vi "unused_getType.vi"(8 "error in (no error)":errorcluster, 11 "Wire in":refnum<class "Wire.lvclass">) -> (0 "error out":errorcluster, 2 "type":refnum<vi>, 3 "Wire out":refnum<class "Wire.lvclass">)   [LabVIEW 2023]
uses:
  Wire.lvclass/Wire.ctl
  Wire.lvclass
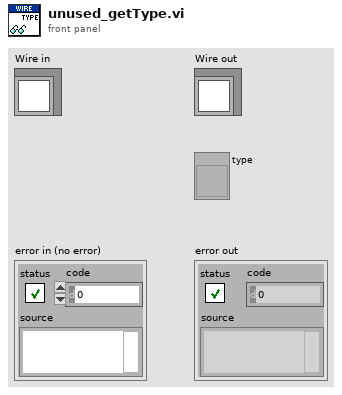
[diagram p1: front panel]
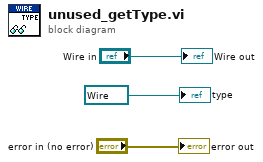
[diagram p0: block diagram]
diagram:
  "error out" <- "error in (no error)"
  "Wire out" <- "Wire in"
  "type" <- refnum<vi> refnum ("type")
